vi "b.vi"(6 "Variant in":variant, 7 "Shift Pressed?":bool, 8 "error in (no error)":errorcluster, 10 "QD Combo Box Ref":refnum<vi>, 11 "QD Launch VI Ref":refnum<vi>) -> (0 "error out":errorcluster, 4 "Variant out":variant)   [LabVIEW 2009]
panel:
  in  "Undo Name":string="VI Server Rename"
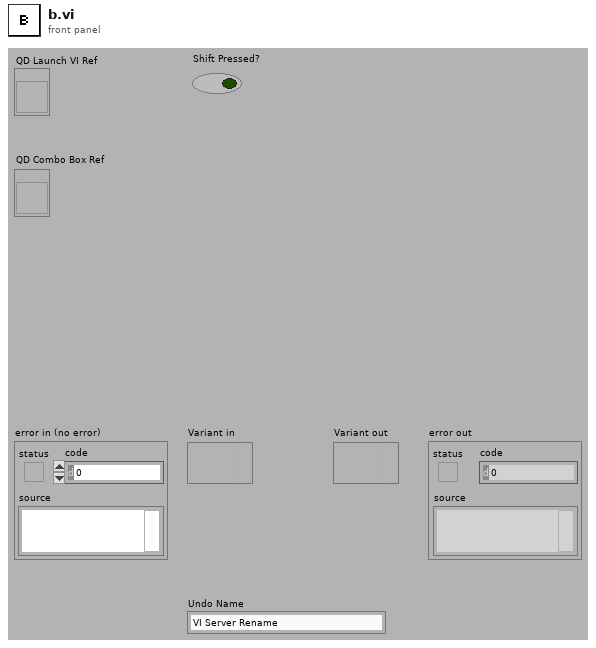
[diagram p1: front panel]
types:
  T1 = typedef "LVRectTypeDef.ctl" = cluster{"left":i16, "top":i16, "right":i16, "bottom":i16}
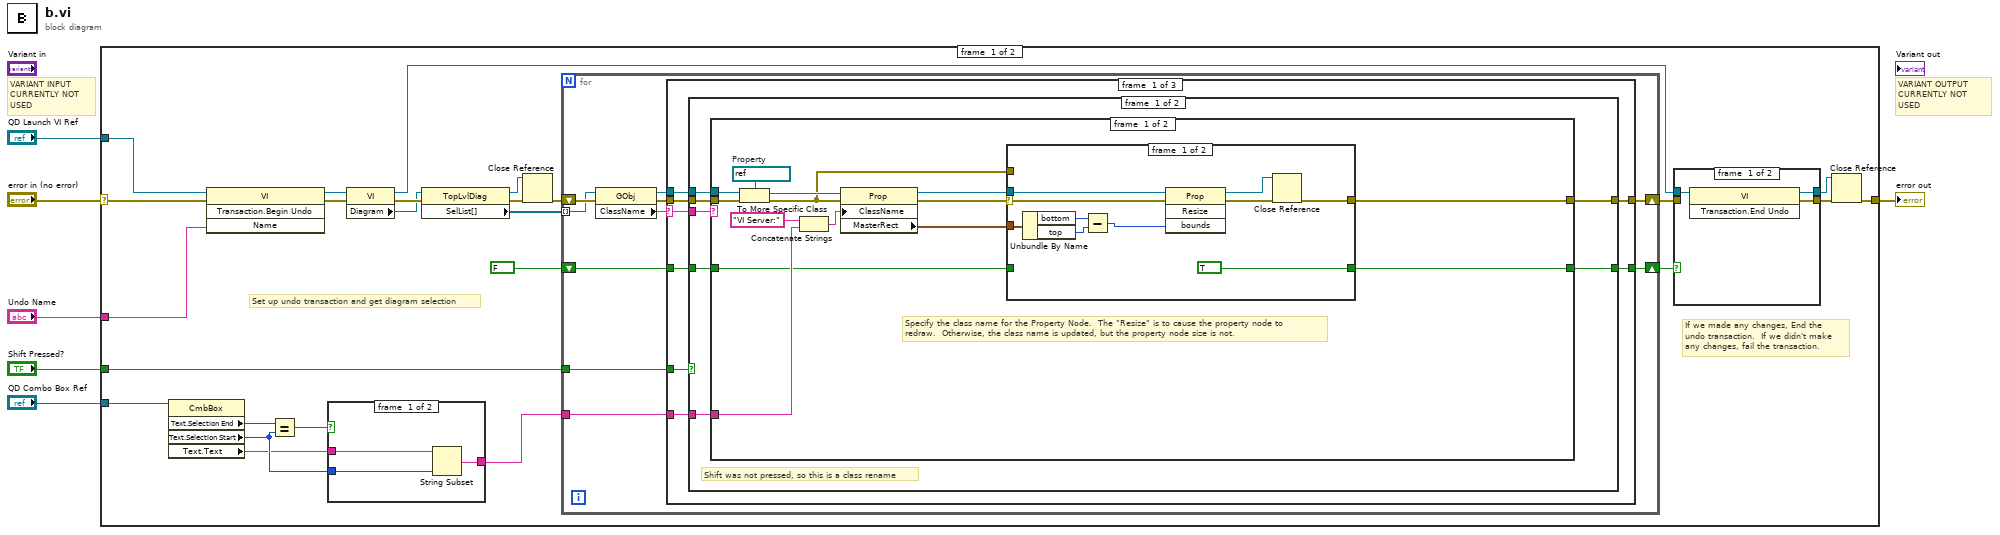
[diagram p0: block diagram]
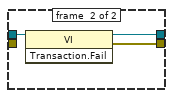
[diagram p3: hidden frame]
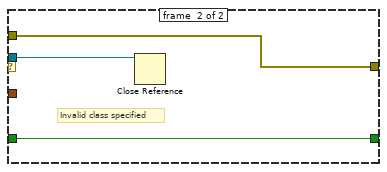
[diagram p4: hidden frame]
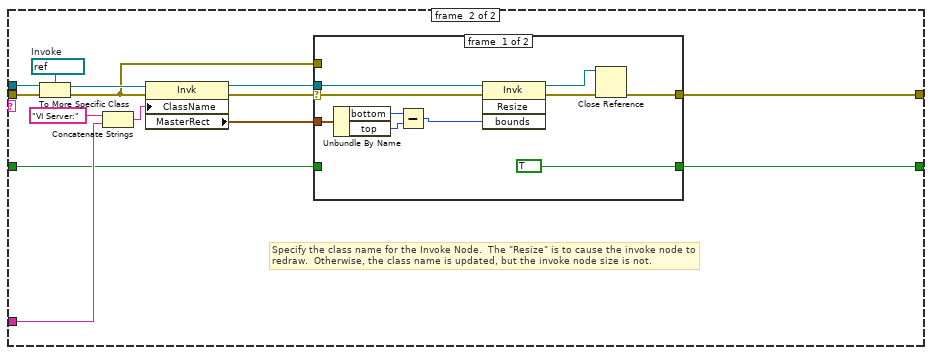
[diagram p5: hidden frame]
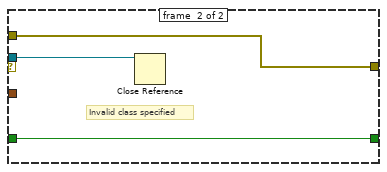
[diagram p6: hidden frame]
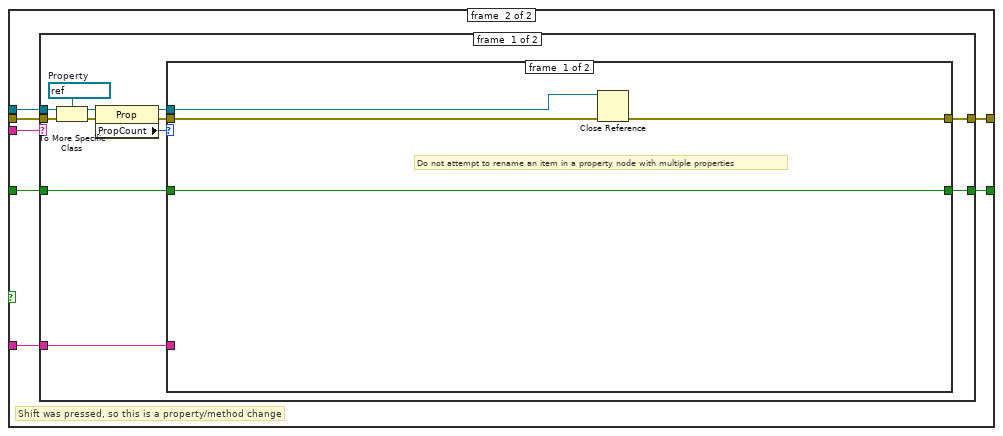
[diagram p7: hidden frame]
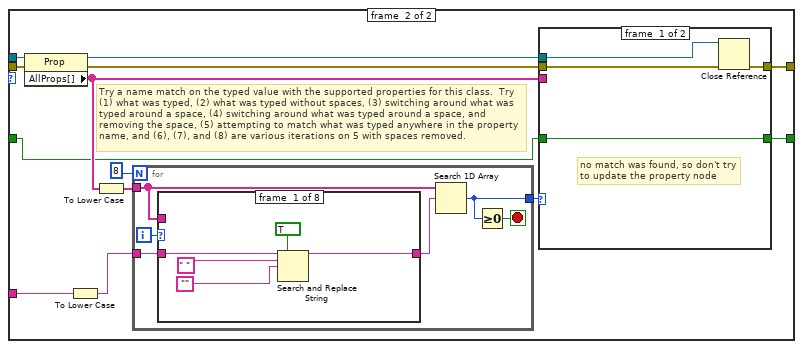
[diagram p8: hidden frame]
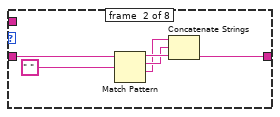
[diagram p9: hidden frame]
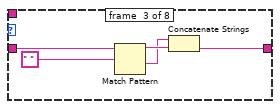
[diagram p10: hidden frame]
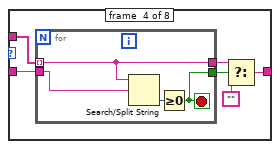
[diagram p11: hidden frame]
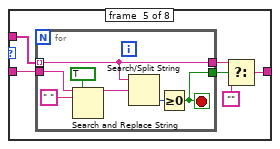
[diagram p12: hidden frame]
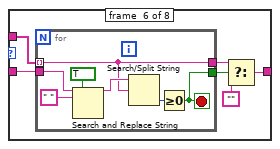
[diagram p13: hidden frame]
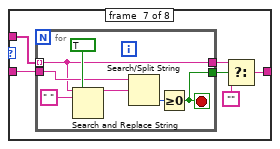
[diagram p14: hidden frame]
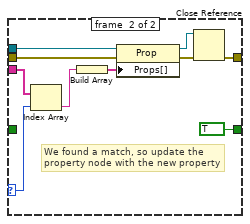
[diagram p16: hidden frame]
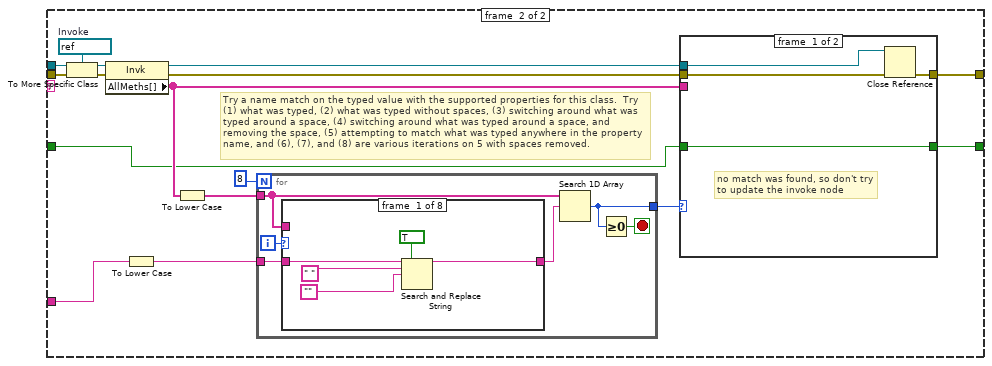
[diagram p17: hidden frame]
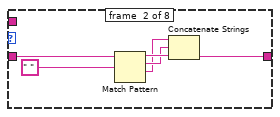
[diagram p18: hidden frame]
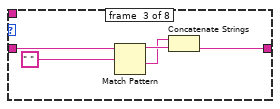
[diagram p19: hidden frame]
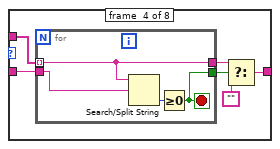
[diagram p20: hidden frame]
diagram:
  # "VARIANT INPUT\nCURRENTLY NOT\nUSED"
  # "VARIANT OUTPUT\nCURRENTLY NOT\nUSED"
  n1 = case shown="No Error" "error in (no error)" {
    selector: "error in (no error)" -> [w14 w364]
    tunnel: [w17 w364] -> w5
    tunnel: "Shift Pressed?" -> [w21 _]
    tunnel: "Undo Name" -> [w31 _]
    tunnel: "QD Launch VI Ref" -> [w13 _]
    tunnel: "QD Combo Box Ref" -> [w8 _]
    frame #0 {
      # "If we made any changes, End the\nundo transaction.  If we didn't make\nany changes, fail the transaction."
      # "Set up undo transaction and get diagram selection"
      n2 = property on="Property Node" class="CmbBox"(reference=w8) -> ("Text.Selection End"=w12:u32, "Text.Selection Start"=w10:u32, "Text.Text"=w9:string)  [unwired: 1 in, 2 out]
      n3 = invoke class="VI" method="Transaction.Begin Undo"(reference=w13, error in=w14, "Name"=w31) -> (reference out=w29:refnum<vi>, error out=w30:errorcluster)  [unwired: 1 in, 2 out]
      n4 = Equal?(x=w12, y=w10) -> (x = y?=w11:bool)
      n5 = case shown="False" w11 {
        tunnel: [w34 w35] -> w7
        tunnel: w10 -> [w33 _]
        tunnel: w9 -> [w32 w35]
        frame #0 {
          n6 = String Subset(string=w32, length (rest)=w33) -> (substring=w34:string)  [unwired: 1 out]
        }
        frame #1 {
        }
      }
      n7 = property class="VI"(reference=w29, error in=w30) -> (reference out=w18:refnum<vi>, error out=w28:errorcluster, "Diagram"=w27:refnum<vi>)
      n8 = property class="TopLvlDiag"(reference=w27, error in=w28) -> (reference out=w23:refnum<vi>, error out=w25:errorcluster, "SelList[]"=w22:refnum<vi>[])
      n9 = Close Reference(reference=w23, error in (no error)=w25) -> (error out=w24:errorcluster)
      n10 = for {
        shift-right: [w46] -> w19
        shift-left: w24 -> [w51]
        shift-right: [w44] -> w20
        shift-left: FALSE -> [w45]
        tunnel: w22 -> [w50] mode=indexing
        tunnel: w21 -> [w43]
        tunnel: w7 -> [w42]
        n11 = property class="GObj"(reference=w50, error in=w51) -> (reference out=w47:refnum<vi>, error out=w48:errorcluster, "ClassName"=w49:string)
        n12 = case shown="\"Invoke\", \"Property\"" w49 {
          selector: w49 -> [w52 _ _]
          tunnel: w48 -> [w56 w353 w363]
          tunnel: w47 -> [w55 w352 w361]
          tunnel: [w53 w347 w362] -> w46
          tunnel: w45 -> [w57 w344 w360]
          tunnel: [w54 w345 w360] -> w44
          tunnel: w43 -> [w58 _ _]
          tunnel: w42 -> [w59 w350 _]
          frame #0 {
            n13 = case shown="True" w58 {
              tunnel: w59 -> [w64 w122]
              tunnel: w57 -> [w60 w124]
              tunnel: w56 -> [w66 w127]
              tunnel: w55 -> [w65 w126]
              tunnel: [w62 w123] -> w54
              tunnel: [w63 w125] -> w53
              tunnel: w52 -> [w61 w121]
              frame #0 {
                # "Shift was not pressed, so this is a class rename"
                n14 = case shown="\"Invoke\"" w61 {
                  tunnel: w66 -> [w80 w107]
                  tunnel: w65 -> [w79 w106]
                  tunnel: w64 -> [w75 w102]
                  tunnel: [w74 w101] -> w63
                  tunnel: [w73 w100] -> w62
                  tunnel: w60 -> [w67 w94]
                  frame #0 {
                    w78 = refnum<vi> refnum  # Property
                    # "Specify the class name for the Property Node.  The \"Resize\" is to cause the property node to\nredraw.  Otherwise, the class name is updated, but the property node size is not."
                    n15 = To More Specific Class(target class=w78, reference=w79, error in=w80) -> (specific class reference=w72:refnum<vi>, error out=w68:errorcluster)
                    n16 = Concatenate Strings("VI Server:" ("string"), w75) -> (w77:string)
                    n17 = property class="Prop"(reference=w72, error in=w68, "ClassName"=w77) -> (reference out=w71:refnum<vi>, error out=w69:errorcluster, "MasterRect"=w70:T1)
                    n18 = case shown="No Error" w69 {
                      selector: w69 -> [w85 _]
                      tunnel: [w90 w93] -> w74
                      tunnel: [TRUE w91] -> w73
                      tunnel: w71 -> [w88 w92]
                      tunnel: w70 -> [w84 _]
                      tunnel: w68 -> [_ w93]
                      tunnel: w67 -> [_ w91]
                      frame #0 {
                        n19 = Unbundle By Name(w84) -> ("bottom"=w83:i16, "top"=w82:i16)
                        n20 = Subtract(x=w83, y=w82) -> (x-y=w81:i16)
                        n21 = invoke class="Prop" method="Resize"(reference=w88, error in=w85, "bounds"=w81) -> (reference out=w86:refnum<vi>, error out=w87:errorcluster)  [unwired: 1 in, 2 out]
                        n22 = Close Reference(reference=w86, error in (no error)=w87) -> (error out=w90:errorcluster)
                      }
                      frame #1 {
                        # "Invalid class specified"
                        n23 = Close Reference(reference=w92) -> ()  [unwired: 1 in, 1 out]
                      }
                    }
                  }
                  frame #1 {
                    w105 = refnum<vi> refnum  # Invoke
                    # "Specify the class name for the Invoke Node.  The \"Resize\" is to cause the invoke node to\nredraw.  Otherwise, the class name is updated, but the invoke node size is not."
                    n24 = To More Specific Class(target class=w105, reference=w106, error in=w107) -> (specific class reference=w99:refnum<vi>, error out=w95:errorcluster)
                    n25 = Concatenate Strings("VI Server:" ("string"), w102) -> (w104:string)
                    n26 = property class="Invk"(reference=w99, error in=w95, "ClassName"=w104) -> (reference out=w98:refnum<vi>, error out=w96:errorcluster, "MasterRect"=w97:T1)
                    n27 = case shown="No Error" w96 {
                      selector: w96 -> [w112 _]
                      tunnel: [w117 w120] -> w101
                      tunnel: [TRUE w118] -> w100
                      tunnel: w98 -> [w115 w119]
                      tunnel: w97 -> [w109 _]
                      tunnel: w95 -> [_ w120]
                      tunnel: w94 -> [_ w118]
                      frame #0 {
                        n28 = Unbundle By Name(w109) -> ("bottom"=w111:i16, "top"=w110:i16)
                        n29 = Subtract(x=w111, y=w110) -> (x-y=w108:i16)
                        n30 = invoke class="Invk" method="Resize"(reference=w115, error in=w112, "bounds"=w108) -> (reference out=w113:refnum<vi>, error out=w114:errorcluster)  [unwired: 1 in, 2 out]
                        n31 = Close Reference(reference=w113, error in (no error)=w114) -> (error out=w117:errorcluster)
                      }
                      frame #1 {
                        # "Invalid class specified"
                        n32 = Close Reference(reference=w119) -> ()  [unwired: 1 in, 1 out]
                      }
                    }
                  }
                }
              }
              frame #1 {
                # "Shift was pressed, so this is a property/method change"
                n33 = case shown="\"Invoke\"" w121 {
                  tunnel: w127 -> [w138 w257]
                  tunnel: w126 -> [w137 w256]
                  tunnel: [w136 w255] -> w125
                  tunnel: w124 -> [w130 w247]
                  tunnel: [w129 w254] -> w123
                  tunnel: w122 -> [w128 w253]
                  frame #0 {
                    w139 = refnum<vi> refnum  # Property
                    n34 = To More Specific Class(target class=w139, reference=w137, error in=w138) -> (specific class reference=w135:refnum<vi>, error out=w134:errorcluster)
                    n35 = property class="Prop"(reference=w135, error in=w134) -> (reference out=w131:refnum<vi>, error out=w132:errorcluster, "PropCount"=w133:i32)
                    n36 = case shown="1" w133 {
                      tunnel: w128 -> [_ w154]
                      tunnel: [w140 w153] -> w136
                      tunnel: w132 -> [w143 w156]
                      tunnel: w131 -> [w142 w155]
                      tunnel: w130 -> [w141 w148]
                      tunnel: [w141 w150] -> w129
                      frame #0 {
                        # "Do not attempt to rename an item in a property node with multiple properties"
                        n37 = Close Reference(reference=w142, error in (no error)=w143) -> (error out=w140:errorcluster)
                      }
                      frame #1 {
                        # "Try a name match on the typed value with the supported properties for this class.  Try (1) what was typed, (2) what was typed without spaces, (3) switching around what was typed around a space, (4) switching around what was typed around a space, and removing the space, (5) attempting to match what was typed anywhere in the property name, and (6), (7), and (8) are various iterations on 5 with spaces removed."
                        n38 = property class="Prop"(reference=w155, error in=w156) -> (reference out=w151:refnum<vi>, error out=w152:errorcluster, "AllProps[]"=w149:string[])
                        n39 = To Lower Case(string=w154) -> (all lower case string=w145:string)
                        n40 = To Lower Case(string=w149) -> (all lower case string=w146:string[])
                        n41 = for {
                          N: 8 -> [_]
                          tunnel: w146 -> [w157]
                          tunnel: [w162] -> w147
                          tunnel: w145 -> [w160]
                          i -> [w159]
                          stop <- w161 stop-if-true
                          n42 = case shown="4" w159 {
                            tunnel: w160 -> [w166 w173 w178 w183 w193 w206 w219 w228]
                            tunnel: [w167 w170 w175 w180 w190 w203 w216 w228] -> w158
                            tunnel: w157 -> [_ _ _ w184 w194 w207 w220 _]
                            frame #0 {
                              n43 = Search and Replace String(replace all?=TRUE ("replace all? (F)"), input string=w166, search string=" ", replace string="") -> (result string=w167:string)  [unwired: 4 in, 3 out]
                            }
                            frame #1 {
                              n44 = Match Pattern(string=w173, regular expression=" ") -> (before substring=w171:string, match substring=w169:string, after substring=w168:string)  [unwired: 1 in, 1 out]
                              n45 = Concatenate Strings(w168, w169, w171) -> (w170:string)
                            }
                            frame #2 {
                              n46 = Match Pattern(string=w178, regular expression=" ") -> (before substring=w176:string, after substring=w174:string)  [unwired: 1 in, 2 out]
                              n47 = Concatenate Strings(w174, w176) -> (w175:string)
                            }
                            frame #3 {
                              n48 = for {
                                tunnel: w184 -> [w185] mode=indexing
                                tunnel: w183 -> [w188]
                                tunnel: [w185] -> w181
                                tunnel: [w186] -> w182
                                stop <- w186 stop-if-true
                                n49 = Search/Split String(string=w185, search string/char (-)=w188) -> (offset of match=w187:i32)  [unwired: 1 in, 2 out]
                                n50 = Greater Or Equal To 0?(x=w187) -> (x >= 0?=w186:bool)
                              }
                              n51 = Select(t=w181, s=w182, f="") -> (s? t:f=w180:string)
                            }
                            frame #4 {
                              n52 = for {
                                tunnel: w194 -> [w197] mode=indexing
                                tunnel: w193 -> [w195]
                                tunnel: [w197] -> w191
                                tunnel: [w200] -> w192
                                stop <- w200 stop-if-true
                                n53 = Search and Replace String(replace all?=TRUE ("replace all? (F)"), input string=w195, search string=" ") -> (result string=w196:string)  [unwired: 5 in, 3 out]
                                n54 = Search/Split String(string=w197, search string/char (-)=w196) -> (offset of match=w201:i32)  [unwired: 1 in, 2 out]
                                n55 = Greater Or Equal To 0?(x=w201) -> (x >= 0?=w200:bool)
                              }
                              n56 = Select(t=w191, s=w192, f="") -> (s? t:f=w190:string)
                            }
                            frame #5 {
                              n57 = for {
                                tunnel: w207 -> [w208] mode=indexing
                                tunnel: w206 -> [w210]
                                tunnel: [w208] -> w204
                                tunnel: [w213] -> w205
                                stop <- w213 stop-if-true
                                n58 = Search and Replace String(replace all?=TRUE ("replace all? (F)"), input string=w210, search string=" ") -> (result string=w209:string)  [unwired: 5 in, 3 out]
                                n59 = Search/Split String(string=w209, search string/char (-)=w208) -> (offset of match=w214:i32)  [unwired: 1 in, 2 out]
                                n60 = Greater Or Equal To 0?(x=w214) -> (x >= 0?=w213:bool)
                              }
                              n61 = Select(t=w204, s=w205, f="") -> (s? t:f=w203:string)
                            }
                            frame #6 {
                              n62 = for {
                                tunnel: w220 -> [w222] mode=indexing
                                tunnel: w219 -> [w223]
                                tunnel: [w222] -> w217
                                tunnel: [w226] -> w218
                                stop <- w226 stop-if-true
                                n63 = Search and Replace String(replace all?=TRUE ("replace all? (F)"), input string=w222, search string=" ") -> (result string=w221:string)  [unwired: 5 in, 3 out]
                                n64 = Search/Split String(string=w223, search string/char (-)=w221) -> (offset of match=w227:i32)  [unwired: 1 in, 2 out]
                                n65 = Greater Or Equal To 0?(x=w227) -> (x >= 0?=w226:bool)
                              }
                              n66 = Select(t=w217, s=w218, f="") -> (s? t:f=w216:string)
                            }
                            frame #7 {
                            }
                          }
                          n67 = Search 1D Array(1D array=w157, element=w158) -> (index of element=w162:i32)  [unwired: 1 in]
                          n68 = Greater Or Equal To 0?(x=w162) -> (x >= 0?=w161:bool)
                        }
                        n69 = case shown="Default" w147 {
                          selector: w147 -> [_ w235]
                          tunnel: [w232 w240] -> w153
                          tunnel: w152 -> [w230 w239]
                          tunnel: w151 -> [w229 w238]
                          tunnel: w148 -> [w231 _]
                          tunnel: [w231 TRUE] -> w150
                          tunnel: w149 -> [_ w236]
                          frame #0 {
                            # "no match was found, so don't try\nto update the property node"
                            n70 = Close Reference(reference=w229, error in (no error)=w230) -> (error out=w232:errorcluster)
                          }
                          frame #1 {
                            # "We found a match, so update the\nproperty node with the new property"
                            n71 = Index Array(array=w236, index=w235) -> (element=w234:string)
                            n72 = Build Array(w234) -> (w233:string[])
                            n73 = property class="Prop"(reference=w238, error in=w239, "Props[]"=w233) -> (reference out=w241:refnum<vi>, error out=w242:errorcluster)
                            n74 = Close Reference(reference=w241, error in (no error)=w242) -> (error out=w240:errorcluster)
                          }
                        }
                      }
                    }
                  }
                  frame #1 {
                    w258 = refnum<vi> refnum  # Invoke
                    # "Try a name match on the typed value with the supported properties for this class.  Try (1) what was typed, (2) what was typed without spaces, (3) switching around what was typed around a space, (4) switching around what was typed around a space, and removing the space, (5) attempting to match what was typed anywhere in the property name, and (6), (7), and (8) are various iterations on 5 with spaces removed."
                    n75 = To More Specific Class(target class=w258, reference=w256, error in=w257) -> (specific class reference=w251:refnum<vi>, error out=w252:errorcluster)
                    n76 = property class="Invk"(reference=w251, error in=w252) -> (reference out=w249:refnum<vi>, error out=w250:errorcluster, "AllMeths[]"=w248:string[])
                    n77 = To Lower Case(string=w253) -> (all lower case string=w244:string)
                    n78 = To Lower Case(string=w248) -> (all lower case string=w245:string[])
                    n79 = for {
                      N: 8 -> [_]
                      tunnel: w245 -> [w259]
                      tunnel: [w264] -> w246
                      tunnel: w244 -> [w262]
                      i -> [w261]
                      stop <- w263 stop-if-true
                      n80 = case shown="4" w261 {
                        tunnel: w262 -> [w268 w275 w280 w285 w295 w308 w321 w330]
                        tunnel: [w269 w272 w277 w282 w292 w305 w318 w330] -> w260
                        tunnel: w259 -> [_ _ _ w286 w296 w309 w322 _]
                        frame #0 {
                          n81 = Search and Replace String(replace all?=TRUE ("replace all? (F)"), input string=w268, search string=" ", replace string="") -> (result string=w269:string)  [unwired: 4 in, 3 out]
                        }
                        frame #1 {
                          n82 = Match Pattern(string=w275, regular expression=" ") -> (before substring=w273:string, match substring=w271:string, after substring=w270:string)  [unwired: 1 in, 1 out]
                          n83 = Concatenate Strings(w270, w271, w273) -> (w272:string)
                        }
                        frame #2 {
                          n84 = Match Pattern(string=w280, regular expression=" ") -> (before substring=w278:string, after substring=w276:string)  [unwired: 1 in, 2 out]
                          n85 = Concatenate Strings(w276, w278) -> (w277:string)
                        }
                        frame #3 {
                          n86 = for {
                            tunnel: w286 -> [w287] mode=indexing
                            tunnel: w285 -> [w290]
                            tunnel: [w287] -> w283
                            tunnel: [w288] -> w284
                            stop <- w288 stop-if-true
                            n87 = Search/Split String(string=w287, search string/char (-)=w290) -> (offset of match=w289:i32)  [unwired: 1 in, 2 out]
                            n88 = Greater Or Equal To 0?(x=w289) -> (x >= 0?=w288:bool)
                          }
                          n89 = Select(t=w283, s=w284, f="") -> (s? t:f=w282:string)
                        }
                        frame #4 {
                          n90 = for {
                            tunnel: w296 -> [w299] mode=indexing
                            tunnel: w295 -> [w297]
                            tunnel: [w299] -> w293
                            tunnel: [w302] -> w294
                            stop <- w302 stop-if-true
                            n91 = Search and Replace String(replace all?=TRUE ("replace all? (F)"), input string=w297, search string=" ") -> (result string=w298:string)  [unwired: 5 in, 3 out]
                            n92 = Search/Split String(string=w299, search string/char (-)=w298) -> (offset of match=w303:i32)  [unwired: 1 in, 2 out]
                            n93 = Greater Or Equal To 0?(x=w303) -> (x >= 0?=w302:bool)
                          }
                          n94 = Select(t=w293, s=w294, f="") -> (s? t:f=w292:string)
                        }
                        frame #5 {
                          n95 = for {
                            tunnel: w309 -> [w310] mode=indexing
                            tunnel: w308 -> [w312]
                            tunnel: [w310] -> w306
                            tunnel: [w315] -> w307
                            stop <- w315 stop-if-true
                            n96 = Search and Replace String(replace all?=TRUE ("replace all? (F)"), input string=w312, search string=" ") -> (result string=w311:string)  [unwired: 5 in, 3 out]
                            n97 = Search/Split String(string=w311, search string/char (-)=w310) -> (offset of match=w316:i32)  [unwired: 1 in, 2 out]
                            n98 = Greater Or Equal To 0?(x=w316) -> (x >= 0?=w315:bool)
                          }
                          n99 = Select(t=w306, s=w307, f="") -> (s? t:f=w305:string)
                        }
                        frame #6 {
                          n100 = for {
                            tunnel: w322 -> [w324] mode=indexing
                            tunnel: w321 -> [w325]
                            tunnel: [w324] -> w319
                            tunnel: [w328] -> w320
                            stop <- w328 stop-if-true
                            n101 = Search and Replace String(replace all?=TRUE ("replace all? (F)"), input string=w324, search string=" ") -> (result string=w323:string)  [unwired: 5 in, 3 out]
                            n102 = Search/Split String(string=w325, search string/char (-)=w323) -> (offset of match=w329:i32)  [unwired: 1 in, 2 out]
                            n103 = Greater Or Equal To 0?(x=w329) -> (x >= 0?=w328:bool)
                          }
                          n104 = Select(t=w319, s=w320, f="") -> (s? t:f=w318:string)
                        }
                        frame #7 {
                        }
                      }
                      n105 = Search 1D Array(1D array=w259, element=w260) -> (index of element=w264:i32)  [unwired: 1 in]
                      n106 = Greater Or Equal To 0?(x=w264) -> (x >= 0?=w263:bool)
                    }
                    n107 = case shown="Default" w246 {
                      selector: w246 -> [_ w336]
                      tunnel: [w334 w341] -> w255
                      tunnel: w250 -> [w332 w340]
                      tunnel: w249 -> [w331 w339]
                      tunnel: w247 -> [w333 _]
                      tunnel: [w333 TRUE] -> w254
                      tunnel: w248 -> [_ w337]
                      frame #0 {
                        # "no match was found, so don't try\nto update the invoke node"
                        n108 = Close Reference(reference=w331, error in (no error)=w332) -> (error out=w334:errorcluster)
                      }
                      frame #1 {
                        # "We found a match, so update the\ninvoke node with the new method"
                        n109 = Index Array(array=w337, index=w336) -> (element=w335:string)
                        n110 = property class="Invk"(reference=w339, error in=w340, "Method"=w335) -> (reference out=w342:refnum<vi>, error out=w343:errorcluster)
                        n111 = Close Reference(reference=w342, error in (no error)=w343) -> (error out=w341:errorcluster)
                      }
                    }
                  }
                }
              }
            }
          }
          frame #1 {
            w354 = refnum<vi> refnum  # ClassSpecifierConstant
            # "Try to change the class of the ClassSpecifierConstant to whatever was typed in Quick Drop.\nIf setting the property returns error 1047, then the specified class name was invalid."
            n112 = To More Specific Class(target class=w354, reference=w352, error in=w353) -> (specific class reference=w351:refnum<vi>, error out=w347:errorcluster)
            n113 = property class="ClassSpecConst"(reference=w351, error in=w347, "Type"=w350) -> (reference out=w348:refnum<vi>, error out=w349:errorcluster)
            n114 = Close Reference(reference=w348, error in (no error)=w349) -> (error out=w346:errorcluster)
            n115 = case shown="False" w344 {
              selector: w344 -> [_ w359]
              tunnel: w346 -> [w358 _]
              tunnel: [w357 w359] -> w345
              frame #0 {
                n116 = Unbundle By Name(w358) -> ("code"=w356:i32)
                n117 = Not Equal?(x=w356, y=1047) -> (x != y?=w357:bool)
              }
              frame #1 {
              }
            }
          }
          frame #2 {
            # "current item is not a Class Specifier Constant, Property Node, or Invoke Node.  Ignore it."
            n118 = Close Reference(reference=w361, error in (no error)=w363) -> (error out=w362:errorcluster)
          }
        }
      }
      n119 = case shown="True" w20 {
        tunnel: w19 -> [_ _]
        tunnel: w18 -> [w38 w41]
        tunnel: [w37 w40] -> w16
        tunnel: [w36 w39] -> w15
        frame #0 {
          n120 = invoke class="VI" method="Transaction.End Undo"(reference=w38) -> (reference out=w36:refnum<vi>, error out=w37:errorcluster)  [unwired: 2 in, 1 out]
        }
        frame #1 {
          n121 = invoke class="VI" method="Transaction.Fail"(reference=w41) -> (reference out=w39:refnum<vi>, error out=w40:errorcluster)  [unwired: 2 in, 1 out]
        }
      }
      n122 = Close Reference(reference=w15, error in (no error)=w16) -> (error out=w17:errorcluster)
    }
    frame #1 {
    }
  }
  "error out" <- w5
